vi "Rd Wr FITS Header JSON.vi"(8 "error in (no error)":errorcluster, 9 "FITS Template":path=path "C:/Users/gsfcprime/Documents/LabVIEW Data/FITS Templates/header0.json", 10 "Write? (F:Read)":bool, 11 "FITS Hdr Rows":T1[](array[typedef])) -> (0 "error out":errorcluster, 3 "FITS Hdr Rows":T1[](array[typedef]))   [LabVIEW 2021]
uses:
  FITS cluster Header Row.ctl
  FITS enum Data Type.ctl
  2e80df6d-94aa-46b9-8b94-ceea8c057880.vi
  659fb017-0e9f-42f9-b06e-930303f00cbc.vi
  <vilib>/JDP Science/JSONtext/Find Item.vi
  <vilib>/JDP Science/JSONtext/Next JSON Value.vi
  <vilib>/JDP Science/JSONtext/String Subset.vi
  <vilib>/JDP Science/JSONtext/Parsing/Advance past next JSON Value (inlined COPY).vi
  <vilib>/JDP Science/JSONtext/Parsing/Advance past whitespace.vi
  <vilib>/JDP Science/JSONtext/Parsing/Advance past String.vi
  <vilib>/JDP Science/JSONtext/Parsing/Advance past Number.vi
  <vilib>/JDP Science/JSONtext/Parsing/Advance past Line Ending.vi
  <vilib>/JDP Science/JSONtext/Parsing/Parse Full Path or Item Name.vi
  <vilib>/JDP Science/JSONtext/Parsing/Advance past Array.vi
  <vilib>/JDP Science/JSONtext/Parsing/Advance past Object.vi
  <vilib>/JDP Science/JSONtext/support/Error Cluster From Code.vi
  <vilib>/JDP Science/JSONtext/Offset/Find Item Locations by Path.vi
  <vilib>/JDP Science/JSONtext/JSON text to Variant.vi
  <vilib>/JDP Science/JSONtext/Variant to JSON Text.vi
  <vilib>/JDP Science/JSONtext/Set Item.vi
  <vilib>/JDP Science/JSONtext/LVClass Serializer/JSONtext LVClass Serializer.lvclass
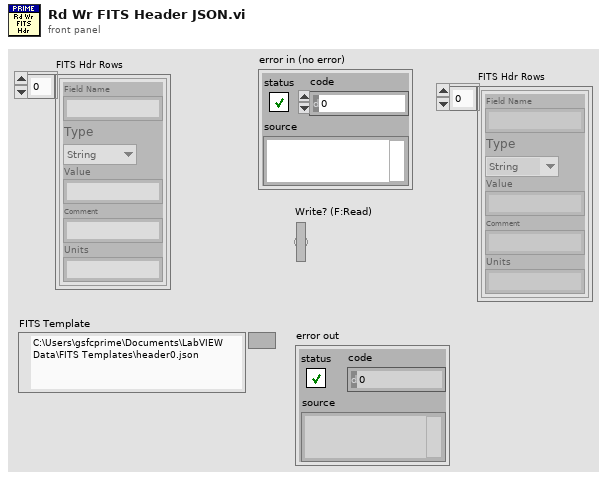
[diagram p1: front panel]
types:
  T1 = typedef "FITS cluster Header Row.ctl" = cluster{"Field Name":string, "Type":T2, "Value":string, "Comment":string, "Units":string}
  T2 = typedef "FITS enum Data Type.ctl" = enum16{"String", "Integer", "Float"}
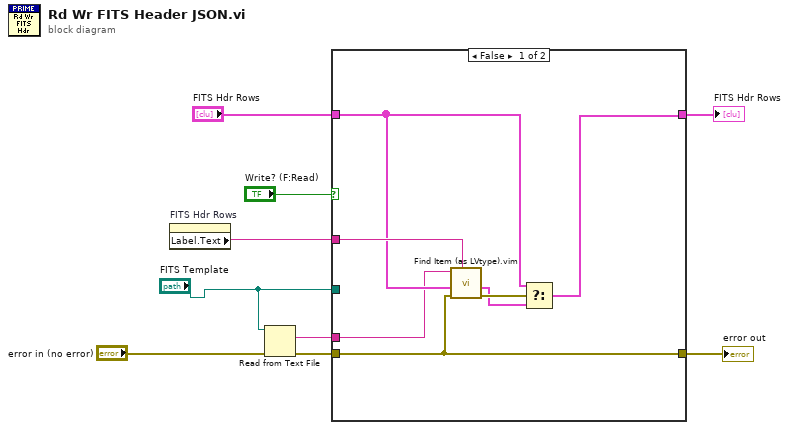
[diagram p0: block diagram]
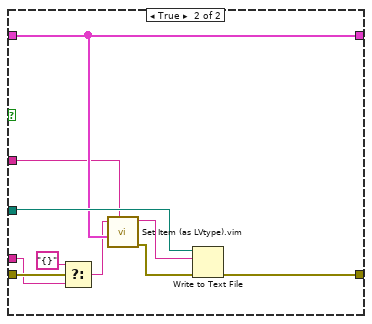
[diagram p2: hidden frame]
diagram:
  n1 = property on="FITS Hdr Rows" class="Arr (strict)"() -> ("Label.Text"=w2:string)  [unwired: 2 in, 2 out]
  n2 = Read from Text File(file (use dialog)="FITS Template", error in="error in (no error)") -> (text=w3:string, error out=w4:errorcluster)  [unwired: 2 in, 2 out]
  n3 = case shown="False" "Write? (F:Read)" {
    tunnel: w4 -> [w10 w21]
    tunnel: "FITS Hdr Rows" -> [w14 w24]
    tunnel: "FITS Template" -> [_ w26]
    tunnel: [w10 w25] -> w6
    tunnel: [w16 w24] -> w5
    tunnel: w2 -> [w15 w23]
    tunnel: w3 -> [w11 w19]
    frame False {
      n4 = call "Find Item (as LVtype).vim"("$Path or Item Name"=w15, "error in (no error)"=w10, "Data Type and Default Value"=w14, "JSON"=w11) -> ("error out"=w13:errorcluster, "Data"=w12:T1[])  [unwired: 4 in, 2 out]
      n5 = Select(t=w14, s=w13, f=w12) -> (s? t:f=w16:T1[])
    }
    frame True {
      n6 = Select(t="{}" ("JSON"), s=w21, f=w19) -> (s? t:f=w18:string)
      n7 = call "Set Item (as LVtype).vim"("$Path or Item Name"=w23, "Anything"=w24, "JSON"=w18) -> ("error out"=w17:errorcluster, "<JSON>"=w22:string)  [unwired: 5 in, 1 out]
      n8 = Write to Text File(file (use dialog)=w26, text=w22, error in=w17) -> (error out=w25:errorcluster)  [unwired: 1 in, 2 out]
    }
  }
  "error out" <- w6
  "FITS Hdr Rows" <- w5
